vi "readfile_param.vi"(7 "error in":errorcluster, 8 "index":i32, 9 "file":string="param.txt", 10 "file (use dialog)":path=path "D:/CTA/Data_test/tmp_150") -> (0 "error out":errorcluster={"status"=TRUE, "code"=1, "source"="Read from Text File in readfile_param.vi->clipconf.vi<APPEND>\nall:\\"}, 1 "clipping":i32[](array[numeric]), 2 "attenuation":i32[](array[numeric]), 3 "channel":i32[](array[numeric]))   [LabVIEW 2009]
panel:
  out "array":dbl[][](array[numeric])
  out "text":string
  out "cancelled":bool
  in  "prompt (Open existing file)":string
  out "refnum out":refnum<file>
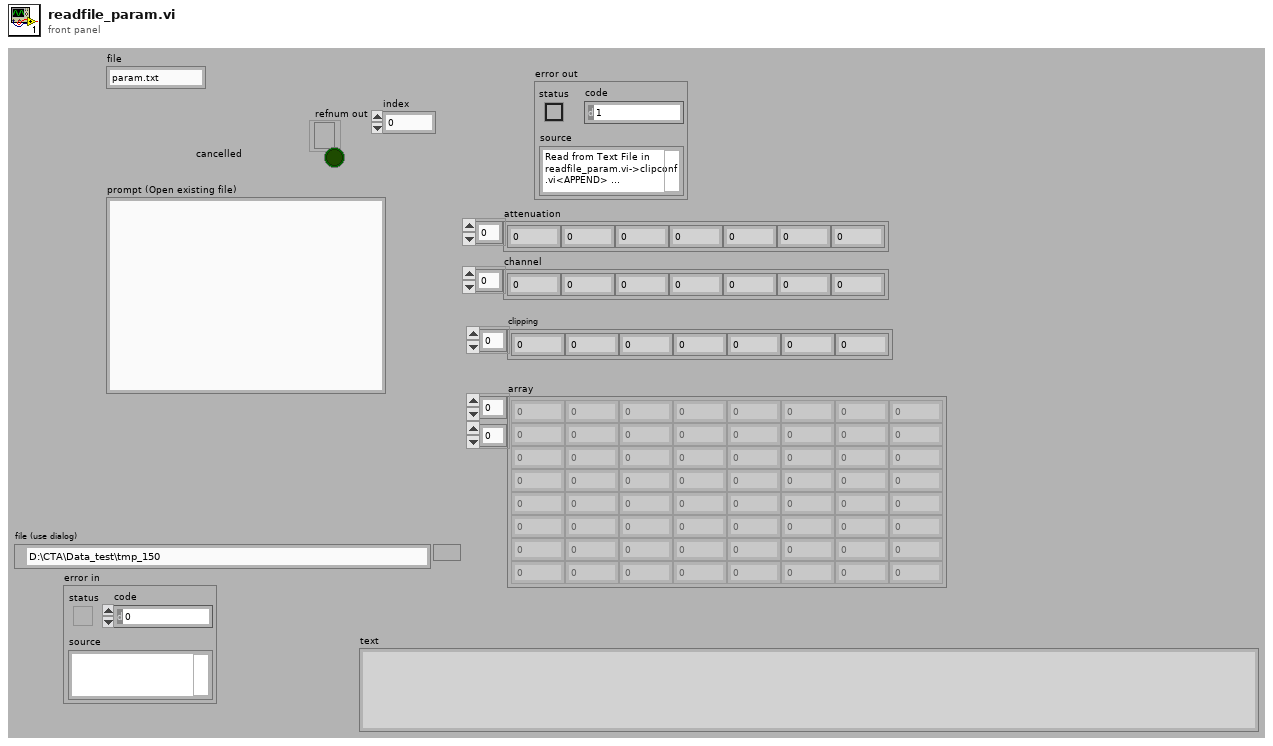
[diagram p1: front panel]
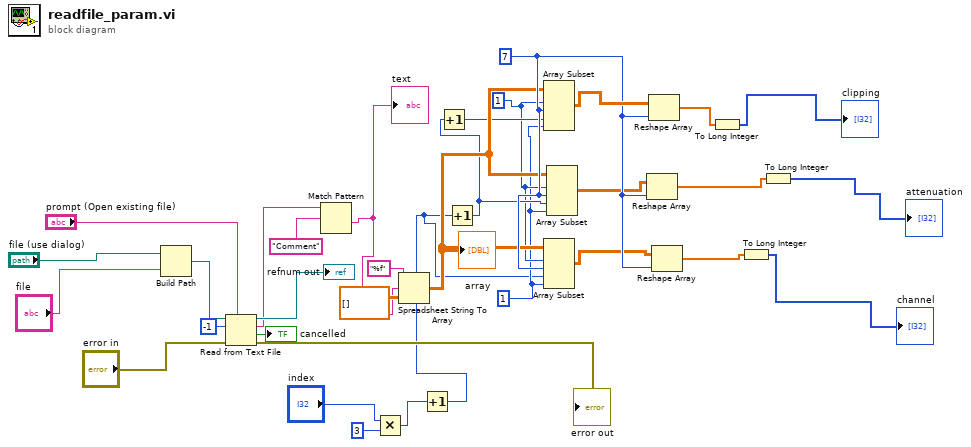
[diagram p0: block diagram]
diagram:
  w11 = 1 ("length")
  w18 = 7 ("length")
  w12 = 1 ("index")
  n1 = Build Path(base path="file (use dialog)", name or relative path="file") -> (appended path=w29:path)
  n2 = Read from Text File(prompt (Open existing file)="prompt (Open existing file)", file (use dialog)=w29, count=-1, error in="error in") -> (refnum out=→"refnum out":refnum<file>, text=w21:string, cancelled=→"cancelled":bool, error out=→"error out":errorcluster)
  n3 = Match Pattern(string=w21, regular expression="Comment") -> (after substring=w20:string)  [unwired: 1 in, 3 out]
  "text" <- w20
  n4 = Multiply(x="index", y=3) -> (x*y=w7:i32)
  n5 = Spreadsheet String To Array(format string="%f", spreadsheet string=w20, array type (2D Dbl)=dbl[][] []) -> (array=w15:dbl[][])  [unwired: 1 in]
  "array" <- w15
  n6 = Increment(x=w7) -> (x+1=w8:i32)
  n7 = Increment(x=w8) -> (x+1=w13:i32)
  n8 = Increment(x=w13) -> (x+1=w14:i32)
  n9 = Array Subset(array=w15, index (row)=w12, length (row)=w18, index (col)=w14, length (col)=w11) -> (w19:dbl[][])
  n10 = Array Subset(array=w15, index (row)=w12, length (row)=w18, index (col)=w8, length (col)=w11) -> (w17:dbl[][])
  n11 = Array Subset(array=w15, index (row)=w12, length (row)=w18, index (col)=w13, length (col)=w11) -> (w16:dbl[][])
  n12 = Reshape Array(w16, w18) -> (w4:dbl[])
  n13 = Reshape Array(w19, w18) -> (w6:dbl[])
  n14 = Reshape Array(w17, w18) -> (w2:dbl[])
  n15 = To Long Integer(number=w6) -> (32bit integer=→"clipping":i32[])
  n16 = To Long Integer(number=w2) -> (32bit integer=→"channel":i32[])
  n17 = To Long Integer(number=w4) -> (32bit integer=→"attenuation":i32[])
